vi "4Pi Obj Lock - 1 Values Organize Plot Data.vi"(0 "Target 01":dbl, 2 "Value Limit":dbl, 7 "Current 2":dbl, 9 "Current 01":dbl, 11 "Stage Pos":dbl) -> (8 "plot value":T1)   [LabVIEW 2016]
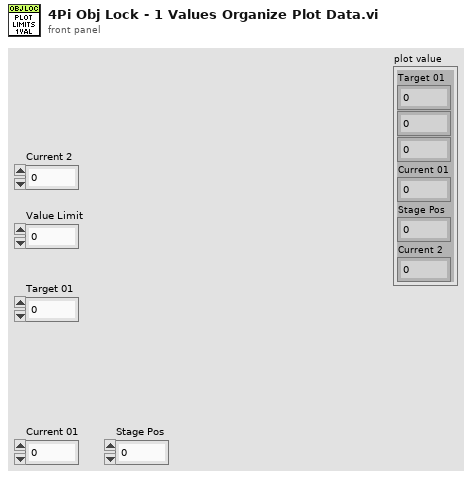
[diagram p1: front panel]
types:
  T1 = cluster{"Target 01":dbl, dbl, dbl, "Current 01":dbl, "Stage Pos":dbl, "Current 2":dbl}
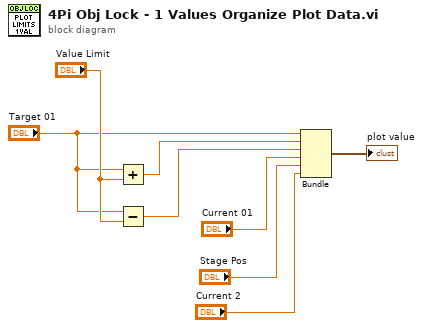
[diagram p0: block diagram]
diagram:
  n1 = Add(x="Target 01", y="Value Limit") -> (x+y=w6:dbl)
  n2 = Subtract(x="Target 01", y="Value Limit") -> (x-y=w5:dbl)
  n3 = Bundle("Target 01"="Target 01", w6, w5, "Current 01"="Current 01", "Stage Pos"="Stage Pos", "Current 2"="Current 2") -> (→"plot value":T1)  [unwired: 1 in]
